vi "Dequeue Beverage.vi"(8 "error in (no error)":errorcluster, 9 "timeout in ms (-1)":i32=-1, 11 "Mock Worker in":refnum<class "Mock Pick Up Order.lvclass">) -> (0 "error out":errorcluster, 1 "timed out?":bool, 2 "Beverage":refnum<class "Beverage.lvclass">, 3 "Mock Worker out":refnum<class "Mock Pick Up Order.lvclass">)   [LabVIEW 2020, in "Mock Pick Up Order.lvclass"]
uses:
  Mock Pick Up Order.lvclass
  Support/Beverages/Beverage/Beverage.lvclass
  Mock Pick Up Order.lvclass/Mock Pick Up Order.ctl
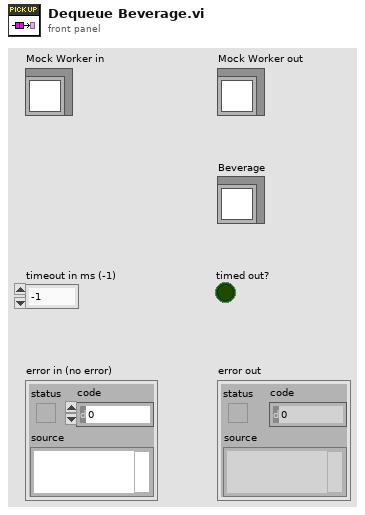
[diagram p1: front panel]
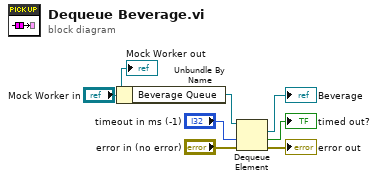
[diagram p0: block diagram]
diagram:
  n1 = Unbundle By Name("Mock Worker in") -> ("Beverage Queue"=w4:refnum<queue>)
  n2 = Dequeue Element(queue=w4, timeout in ms (-1)="timeout in ms (-1)", error in (no error)="error in (no error)") -> (element=→"Beverage":refnum<class "Beverage.lvclass">, timed out?=→"timed out?":bool, error out=→"error out":errorcluster)  [unwired: 1 out]
  "Mock Worker out" <- "Mock Worker in"
